vi "Set Component Settings.vi"(8 "error in (no error)":errorcluster, 9 "component settings":T2[](array[typedef]), 10 "settings id":T1={"plugin"=-1, "thread"=-1, "group"=-1, "transfer"=-1, "channel"=-1}, 11 "framework configuration in":T3) -> (0 "error out":errorcluster, 3 "framework configuration out":T3)   [LabVIEW 2017, in "DSF Core.lvlib"]
uses:
  DSF Core.lvlib
  Typedefs/DSF Engine Framework Configuration.ctl
  Typedefs/DSF Settings Info.ctl
  Typedefs/DSF Engine Plugin Configuration.ctl
  Typedefs/DSF Engine Plugin Thread Configuration.ctl
  Typedefs/DSF Engine Transfer Group Configuration.ctl
  Typedefs/DSF Engine Transfer Configuration.ctl
  Typedefs/DSF Engine Channel Configuration.ctl
  Typedefs/DSF Configuration ID.ctl
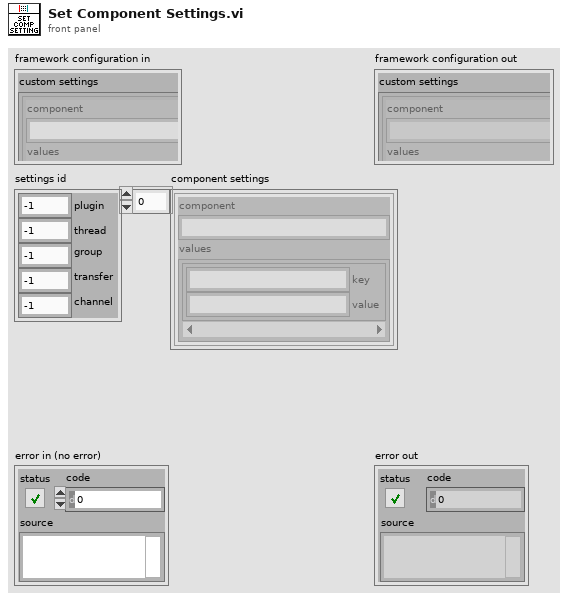
[diagram p1: front panel]
types:
  T1 = typedef "DSF Core.lvlib/DSF Configuration ID.ctl" = cluster{"plugin":i32, "thread":i32, "group":i32, "transfer":i32, "channel":i32}
  T2 = typedef "DSF Core.lvlib/DSF Settings Info.ctl" = cluster{"component":string, "values":cluster{"key":string, "value":string}[]}
  T3 = typedef "DSF Core.lvlib/DSF Engine Framework Configuration.ctl" = cluster{"custom settings":T2[], "plugins":T4[]}
  T4 = typedef "DSF Core.lvlib/DSF Engine Plugin Configuration.ctl" = cluster{"core settings":T2, "component settings":T2[], "threads":T5[]}
  T5 = typedef "DSF Core.lvlib/DSF Engine Plugin Thread Configuration.ctl" = cluster{"core settings":T2, "component settings":T2[], "transfer groups":T6[]}
  T6 = typedef "DSF Core.lvlib/DSF Engine Transfer Group Configuration.ctl" = cluster{"component settings":T2[], "transfers":T7[], "core settings":T2}
  T7 = typedef "DSF Core.lvlib/DSF Engine Transfer Configuration.ctl" = cluster{"core settings":T2, "component settings":T2[], "channels":T8[]}
  T8 = typedef "DSF Core.lvlib/DSF Engine Channel Configuration.ctl" = cluster{"core settings":T2, "component settings":T2[]}
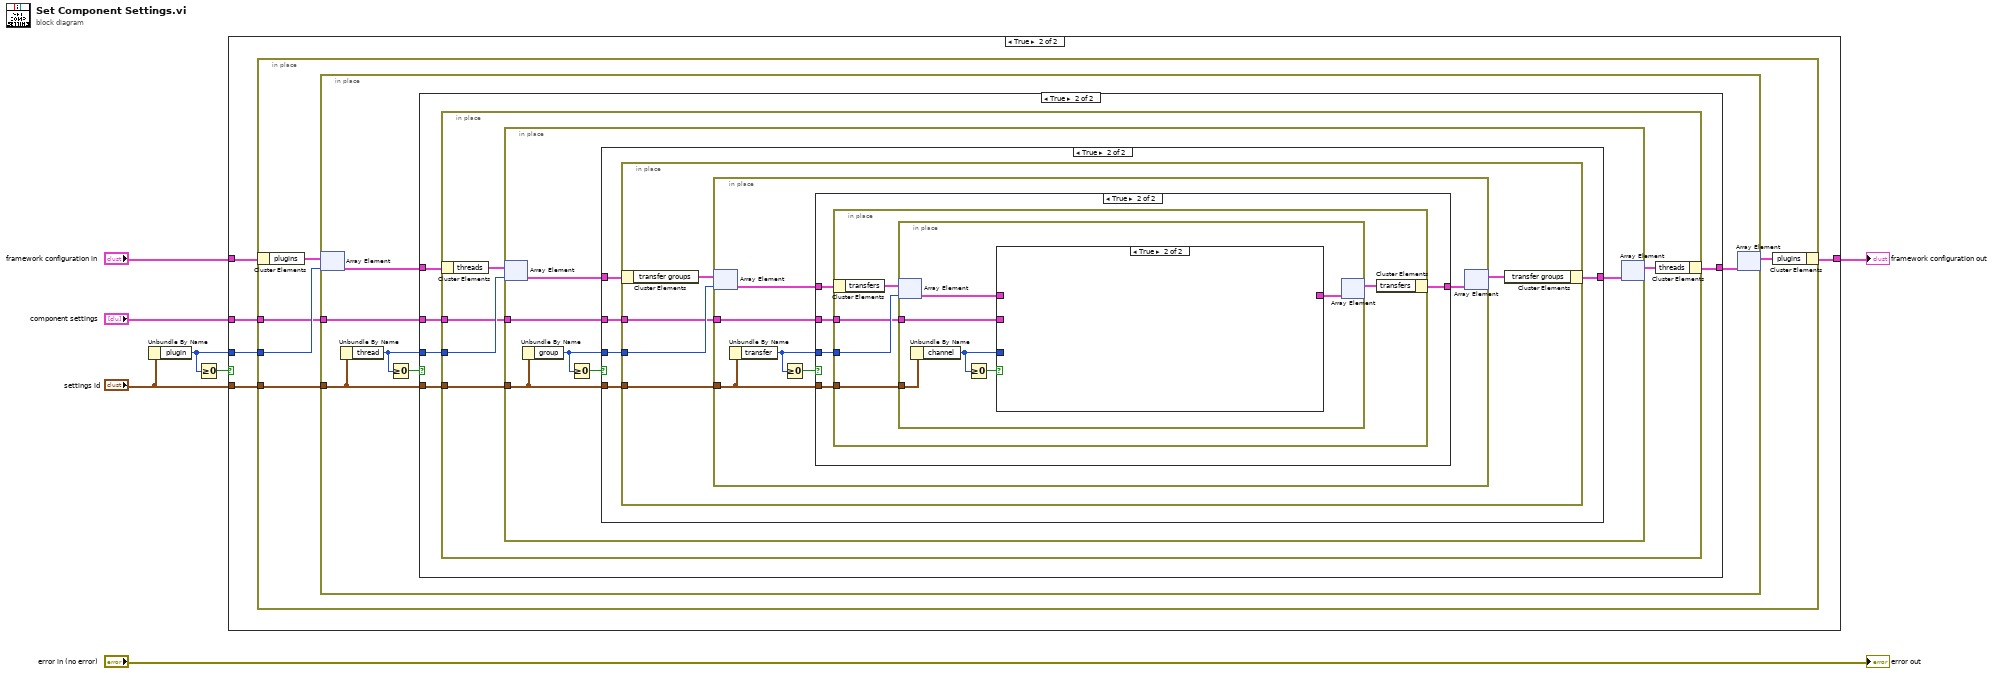
[diagram p0: block diagram]
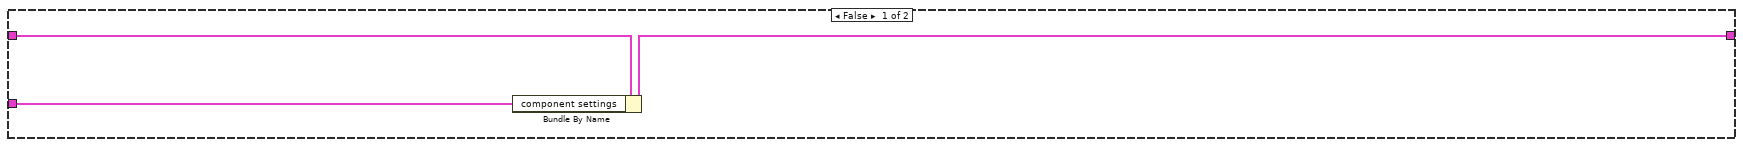
[diagram p3: hidden frame]
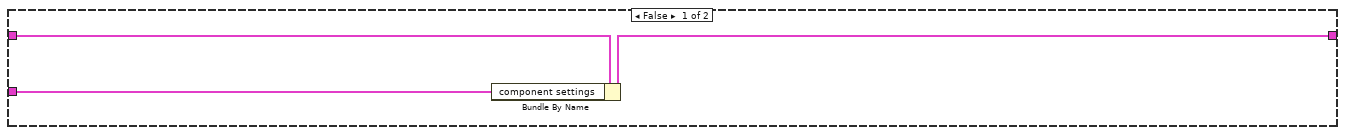
[diagram p4: hidden frame]
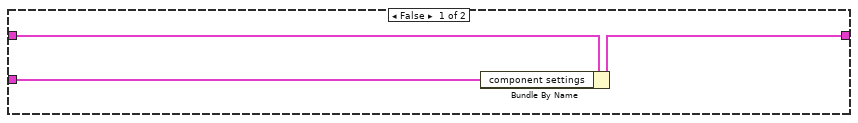
[diagram p5: hidden frame]
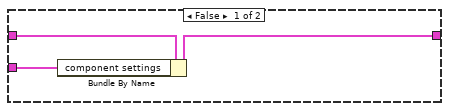
[diagram p6: hidden frame]
diagram:
  n1 = Unbundle By Name("settings id") -> ("plugin"=w6:i32)
  n2 = Greater Or Equal To 0?(x=w6) -> (x >= 0?=w7:bool)
  n3 = case shown="True" w7 {
    tunnel: "settings id" -> [_ w13]
    tunnel: w6 -> [_ w11]
    tunnel: "framework configuration in" -> [w8 w12]
    tunnel: [w8 w10] -> w2
    tunnel: "component settings" -> [_ w9]
    frame False {
    }
    frame True {
      n4 = in-place {
        in-place-border: w13 -> [w18]
        in-place-border: w11 -> [w16]
        in-place-border: w9 -> [w14]
        n5 = in-place-cluster #1(w12) -> ("plugins"=w17:T4[])
        n6 = in-place {
          in-place-border: w18 -> [w23]
          in-place-border: w14 -> [w19]
          n7 = in-place-array #2(w17, w16) -> (w21:T4)
          n8 = Unbundle By Name(w23) -> ("thread"=w22:i32)
          n9 = Greater Or Equal To 0?(x=w22) -> (x >= 0?=w24:bool)
          n10 = case shown="True" w24 {
            tunnel: w23 -> [_ w32]
            tunnel: w22 -> [_ w30]
            tunnel: w21 -> [w26 w31]
            tunnel: [w25 w29] -> w20
            tunnel: w19 -> [w27 w28]
            frame False {
              n11 = Bundle By Name(cluster=w26, "component settings"=w27) -> (w25:T4)
            }
            frame True {
              n12 = in-place {
                in-place-border: w32 -> [w37]
                in-place-border: w30 -> [w35]
                in-place-border: w28 -> [w33]
                n13 = in-place-cluster #3(w31) -> ("threads"=w36:T5[])
                n14 = in-place {
                  in-place-border: w37 -> [w43]
                  in-place-border: w33 -> [w38]
                  n15 = in-place-array #4(w36, w35) -> (w40:T5)
                  n16 = Unbundle By Name(w43) -> ("group"=w41:i32)
                  n17 = Greater Or Equal To 0?(x=w41) -> (x >= 0?=w42:bool)
                  n18 = case shown="True" w42 {
                    tunnel: w43 -> [_ w51]
                    tunnel: w41 -> [_ w49]
                    tunnel: w40 -> [w45 w50]
                    tunnel: [w44 w48] -> w39
                    tunnel: w38 -> [w46 w47]
                    frame False {
                      n19 = Bundle By Name(cluster=w45, "component settings"=w46) -> (w44:T5)
                    }
                    frame True {
                      n20 = in-place {
                        in-place-border: w51 -> [w56]
                        in-place-border: w49 -> [w54]
                        in-place-border: w47 -> [w52]
                        n21 = in-place-cluster #5(w50) -> ("transfer groups"=w55:T6[])
                        n22 = in-place {
                          in-place-border: w56 -> [w62]
                          in-place-border: w52 -> [w57]
                          n23 = in-place-array #6(w55, w54) -> (w59:T6)
                          n24 = Unbundle By Name(w62) -> ("transfer"=w60:i32)
                          n25 = Greater Or Equal To 0?(x=w60) -> (x >= 0?=w61:bool)
                          n26 = case shown="True" w61 {
                            tunnel: w62 -> [_ w70]
                            tunnel: w60 -> [_ w68]
                            tunnel: w59 -> [w64 w69]
                            tunnel: [w63 w67] -> w58
                            tunnel: w57 -> [w65 w66]
                            frame False {
                              n27 = Bundle By Name(cluster=w64, "component settings"=w65) -> (w63:T6)
                            }
                            frame True {
                              n28 = in-place {
                                in-place-border: w70 -> [w75]
                                in-place-border: w68 -> [w73]
                                in-place-border: w66 -> [w71]
                                n29 = in-place-cluster #7(w69) -> ("transfers"=w74:T7[])
                                n30 = in-place {
                                in-place-border: w75 -> [w81]
                                in-place-border: w71 -> [w76]
                                n31 = in-place-array #8(w74, w73) -> (w78:T7)
                                n32 = Unbundle By Name(w81) -> ("channel"=w79:i32)
                                n33 = Greater Or Equal To 0?(x=w79) -> (x >= 0?=w80:bool)
                                n34 = case shown="True" w80 {
                                tunnel: w79 -> [_ w85]
                                tunnel: w78 -> [w84 w88]
                                tunnel: [w83 w86] -> w77
                                tunnel: w76 -> [w82 w87]
                                frame False {
                                n35 = Bundle By Name(cluster=w84, "component settings"=w82) -> (w83:T7)
                                }
                                frame True {
                                n36 = in-place {
                                in-place-border: w87 -> [w89]
                                in-place-border: w85 -> [w90]
                                n37 = in-place-cluster #9(w88) -> ("channels"=w92:T8[])
                                n38 = in-place {
                                in-place-border: w89 -> [w94]
                                n39 = in-place-array #10(w92, w90) -> (w95:T8)
                                n40 = Bundle By Name(cluster=w95, "component settings"=w94) -> (w93:T8)
                                n41 = in-place-array #10(w93) -> (w91:T8[])  [unwired: 1 out]
                                }
                                n42 = in-place-cluster #9("channels"=w91) -> (w86:T7)
                                }
                                }
                                }
                                n43 = in-place-array #8(w77) -> (w72:T7[])  [unwired: 1 out]
                                }
                                n44 = in-place-cluster #7("transfers"=w72) -> (w67:T6)
                              }
                            }
                          }
                          n45 = in-place-array #6(w58) -> (w53:T6[])  [unwired: 1 out]
                        }
                        n46 = in-place-cluster #5("transfer groups"=w53) -> (w48:T5)
                      }
                    }
                  }
                  n47 = in-place-array #4(w39) -> (w34:T5[])  [unwired: 1 out]
                }
                n48 = in-place-cluster #3("threads"=w34) -> (w29:T4)
              }
            }
          }
          n49 = in-place-array #2(w20) -> (w15:T4[])  [unwired: 1 out]
        }
        n50 = in-place-cluster #1("plugins"=w15) -> (w10:T3)
      }
    }
  }
  "framework configuration out" <- w2
  "error out" <- "error in (no error)"
